vi "Round nearest Int to Places.vi"(1 "Places In":i32, 2 "Float In":sgl) -> (0 "Float Out":sgl format="%.4g")   [LabVIEW 2024, in "LVarex.lvlib"]
uses:
  LVarex.lvlib
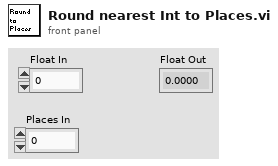
[diagram p1: front panel]
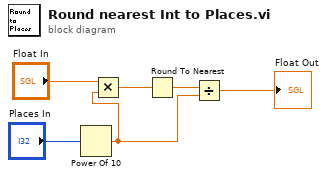
[diagram p0: block diagram]
diagram:
  n1 = Power Of 10(x="Places In") -> (10^x=w2:dbl)
  n2 = Multiply(x="Float In", y=w2) -> (x*y=w4:dbl)
  n3 = Round To Nearest(number=w4) -> (nearest integer value=w3:dbl)
  n4 = Divide(x=w3, y=w2) -> (x/y=→"Float Out":dbl)
